vi "SetBounds.vi"(8 "error in (no error)":errorcluster, 10 "bounds":cluster{"width":u32, "height":u32}, 11 "text item in":refnum<class "text item.lvclass">) -> (0 "error out":errorcluster, 3 "text item out":refnum<class "text item.lvclass">)   [LabVIEW 2009, in "text item.lvclass"]
uses:
  text item.lvclass
  text item.lvclass/text item.ctl
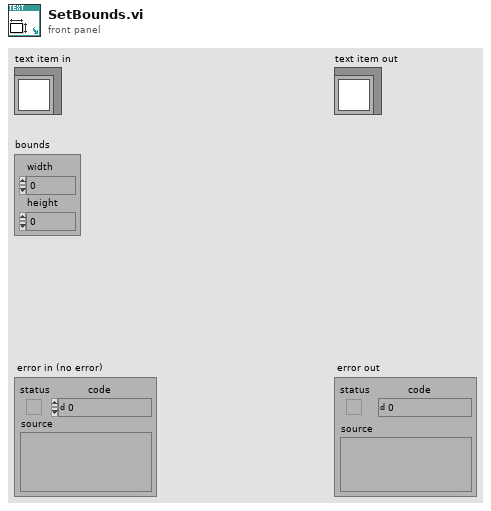
[diagram p1: front panel]
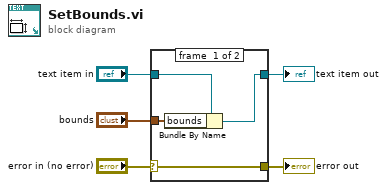
[diagram p0: block diagram]
diagram:
  n1 = case shown="No Error" "error in (no error)" {
    selector: "error in (no error)" -> [w6 w10]
    tunnel: "text item in" -> [w9 w11]
    tunnel: [w8 w11] -> w4
    tunnel: "bounds" -> [w7 _]
    tunnel: [w6 w10] -> w1
    frame #0 {
      n2 = Bundle By Name(cluster=w9, "bounds"=w7) -> (w8:refnum<class "text item.lvclass">)
    }
    frame #1 {
    }
  }
  "error out" <- w1
  "text item out" <- w4
